vi "读二进制文件.vi"() -> ()   [LabVIEW 2015]
panel:
  out "Numeric":dbl
  out "data to file":dbl[](graph)
  out "Array":dbl[](array[numeric])
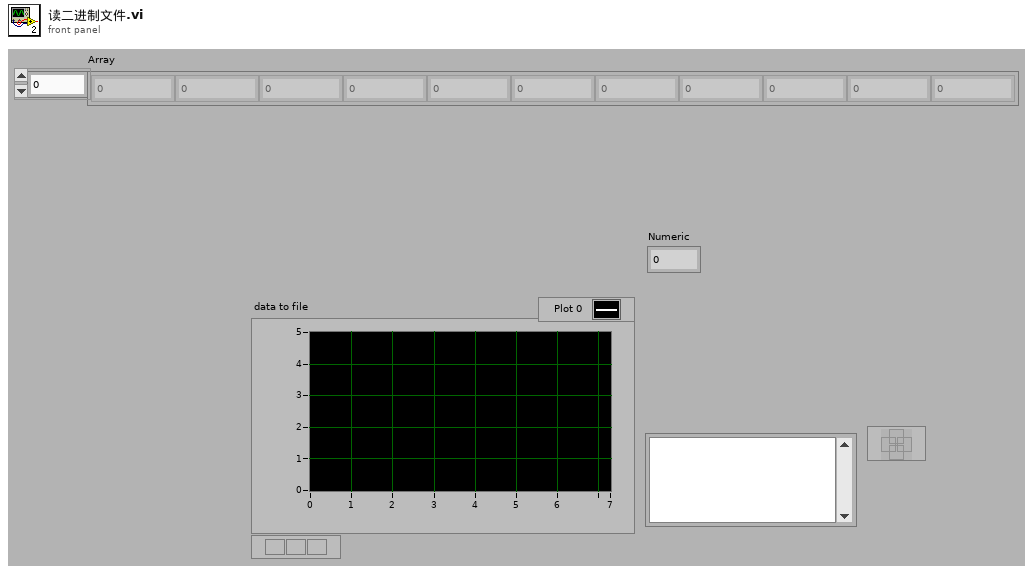
[diagram p1: front panel]
types:
  T1 = enum16{"open", "replace", "create", "open or create", "replace or create", "replace or create with confirmation"}
  T2 = enum16{"big-endian, network order", "native, host order", "little-endian"}
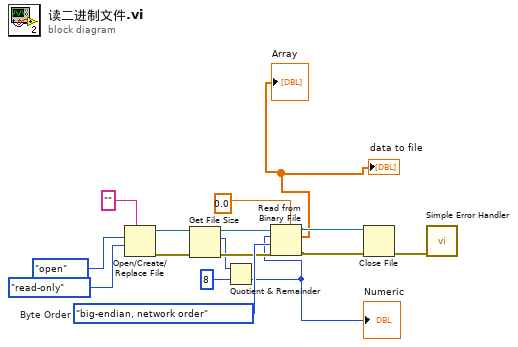
[diagram p0: block diagram]
diagram:
  w13 = T2."big-endian, network order"  # Byte Order
  n1 = Open/Create/Replace File(prompt="", operation (0:open)=T1."open", access (0:read/write)=enum16{"read/write", "read-only", "write-only"}."read-only") -> (refnum out=w9:refnum<file>, error out=w8:errorcluster)  [unwired: 3 in, 1 out]
  n2 = Get File Size(file=w9, error in=w8) -> (refnum out=w7:refnum<file>, size (in bytes)=w5:i64, 0:w6:errorcluster)
  n3 = Quotient & Remainder(x=w5, y=i64 8) -> (floor(x/y)=w2:i64)  [unwired: 1 out]
  "Numeric" <- w2
  n4 = Read from Binary File(5:0.0, 8:w6, 9:w13, 10:w2, 11:w7) -> (0:w12:errorcluster, 2:→"Array" →"data to file":dbl[], 3:w11:refnum<file>)  [unwired: 1 in, 1 out]
  n5 = Close File(refnum=w11, error in=w12) -> (error out=w16:errorcluster)  [unwired: 1 out]
  n6 = call <vilib>:"Simple Error Handler.vi"("error in (no error)"=w16) -> ()  [unwired: 4 in, 5 out]
